vi "Initialise.vi.LOCAL.vi"(8 "error in (no error)":errorcluster, 10 "Message in":refnum<class "InitialiseMessage.lvclass">, 11 "Galvo in":refnum<class "ImagingModeSPIM.lvclass">) -> (0 "error out":errorcluster, 3 "Galvo out":refnum<class "ImagingModeSPIM.lvclass">)   [LabVIEW 2012, in "ImagingModeSPIM.lvclass"]
doc: "This method is called when an initialise message is received. It mainly initialises the RabbitMQ connectivity. \n\nOverride this method when your component needs special initialisation (e.g. of software or hardware resources). In that case, don't forget to call the parent for proper implementation. If your component owns subcomponents, they count as resources, so you have to initialise them by calling their own initialise functions"
uses:
  ImagingModeSPIM.lvclass
  <vilib>/Distrio/Murmex/InitialiseMessage/InitialiseMessage.lvclass
  <vilib>/Distrio/Murmex/Murmex/Murmex.lvclass
  ImagingModeSPIM.lvclass/ImagingModeSPIM.ctl
  <vilib>/Distrio/Murmex/UpdateMessage/UpdateMessage.lvclass
panel:
  # "This method is called when the INTIALISE\ntrigger is sent. \n\nOverride this method when your component needs to\nrespond to this trigger. \n\nCall parent for proper implementation"
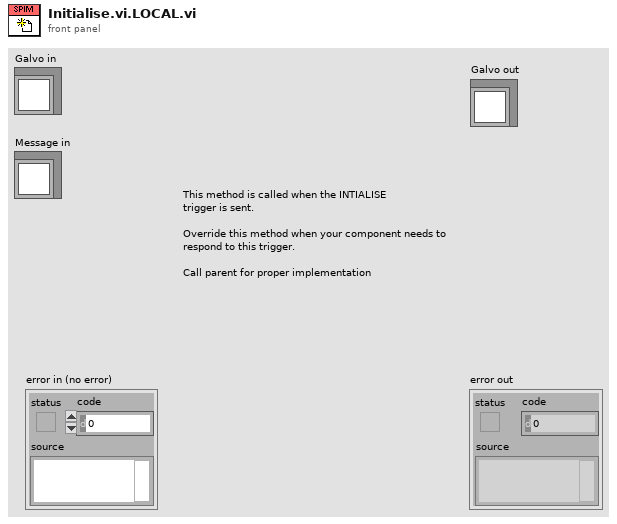
[diagram p1: front panel]
types:
  T1 = enum8{"Enabled", "Disabled", "Disabled and Grayed Out"}
  T2 = typedef "ImagingModeSPIM.lvclass/number of channels.ctl" = enum16{"empty", "double sided + PC", "double sided + WFS"}
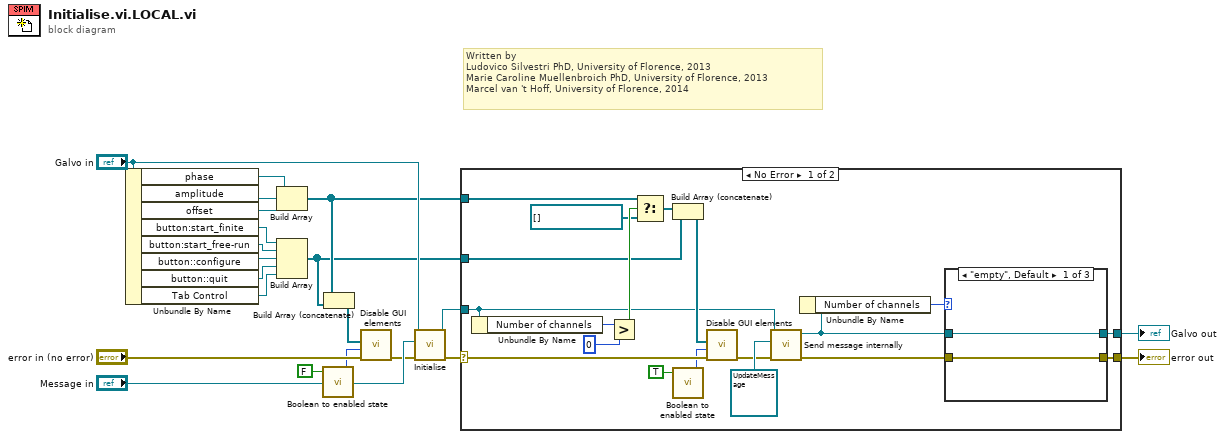
[diagram p0: block diagram]
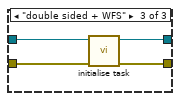
[diagram p3: hidden frame]
diagram:
  # "Written by \nLudovico Silvestri PhD, University of Florence, 2013 \nMarie Caroline Muellenbroich PhD, University of Florence, 2013 \nMarcel van 't Hoff, University of Florence, 2014"
  n1 = Unbundle By Name("Galvo in") -> ("phase"=w11:refnum<vi>, "amplitude"=w10:refnum<vi>, "offset"=w9:refnum<vi>, "button:start_finite"=w8:refnum<vi>, "button:start_free-run"=w7:refnum<vi>, "button::configure"=w6:refnum<vi>, "button::quit"=w5:refnum<vi>, "Tab Control"=w4:refnum<vi>)
  n2 = Build Array(w11, w10, w9) -> (w3:refnum<vi>[])
  n3 = Build Array(w8, w7, w6, w5, w4) -> (w2:refnum<vi>[])
  n4 = call <vilib>:"Boolean to enabled state.vi"("boolean in"=FALSE) -> ("enabled status out"=w12:T1)  [unwired: 4 in]
  n5 = Build Array (concatenate)(w3, w2) -> (w1:refnum<vi>[])
  n6 = call <vilib>:"Disable GUI elements.vi"("error in (no error)"="error in (no error)", "enabled state"=w12, "control refs"=w1) -> ("error out"=w15:errorcluster)  [unwired: 8 in]
  n7 = call-parent "Initialise.vi"("error in (no error)"=w15, "Message in"="Message in", "Murmex in"="Galvo in") -> ("error out"=w17:errorcluster, "Murmex out"=w20:refnum<class "ImagingModeSPIM.lvclass">)  [unwired: 7 in]
  n8 = case shown="No Error" w17 {
    selector: w17 -> [w40 w49]
    tunnel: w20 -> [w28 w50]
    tunnel: [w25 w49] -> w19
    tunnel: [w24 w50] -> w18
    tunnel: w3 -> [w34 _]
    tunnel: w2 -> [w30 _]
    frame No Error {
      n9 = Unbundle By Name(w28) -> ("Number of channels"=w36:T2)
      n10 = Greater?(x=w36, y=u16 0) -> (0:w35:bool)
      n11 = Select(t=w34, s=w35, f=refnum<vi>[] []) -> (s? t:f=w32:refnum<vi>[])
      n12 = Build Array (concatenate)(w32, w30) -> (w31:refnum<vi>[])
      n13 = call <vilib>:"Boolean to enabled state.vi"("boolean in"=TRUE) -> ("enabled status out"=w39:T1)  [unwired: 4 in]
      n14 = call <vilib>:"Disable GUI elements.vi"("error in (no error)"=w40, "enabled state"=w39, "control refs"=w31) -> ("error out"=w27:errorcluster)  [unwired: 8 in]
      n15 = call <vilib>:"Send message internally.vi"("error in (no error)"=w27, "Message"=refnum<class "UpdateMessage.lvclass"> refnum ("Murmex.lvlib:UpdateMessage"), "Murmex in"=w28) -> ("error out"=w26:errorcluster, "Murmex out"=w23:refnum<class "ImagingModeSPIM.lvclass">)  [unwired: 7 in]
      n16 = Unbundle By Name(w23) -> ("Number of channels"=w22:T2)
      n17 = case shown="\"empty\", Default" w22 {
        tunnel: w26 -> [w41 w43 w47]
        tunnel: [w41 w43 w45] -> w25
        tunnel: w23 -> [w42 w44 w48]
        tunnel: [w42 w44 w46] -> w24
        frame "empty", Default {
        }
        frame "double sided + PC" {
        }
        frame "double sided + WFS" {
          n18 = call-dynamic "initialise task.vi"("error in (no error)"=w47, "ImagingModeSPIM in"=w48) -> ("error out"=w45:errorcluster, "ImagingModeSPIM out"=w46:refnum<class "ImagingModeSPIM.lvclass">)  [unwired: 8 in]
        }
      }
    }
    frame Error {
    }
  }
  "error out" <- w19
  "Galvo out" <- w18
